vi "TSP-Link Reset.vi"(8 "error in (no error)":errorcluster, 11 "VISA resource name":refnum<visa-resource-name>) -> (0 "error out":errorcluster, 3 "VISA resource name out":refnum<visa-resource-name>, 4 "Command String":string)   [LabVIEW 2012, in "Keithley 2600 Series.lvlib"]
doc: "Initializes (resets) all nodes (instruments) in the TSP-Link system.\n\nThis VI will erase all knowledge of other nodes connected on the TSP-Link and will regenerate the system configuration. This VI must be called at least once before any remote nodes can be accessed. If the node number for any instrument is changed, the TSP-Link must again be initialized.\n\n<b>Functions and Attributes Used</b>\ntsplink.reset()\n\nNote:\nTSP-Link feature is not supported with Keithley 2604B, 2614B, 2634B."
uses:
  Keithley 2600 Series.lvlib
  Private/GlobalVariables.vi
panel:
  # "(c) 2008 Keithley Instruments, Inc.  ALL RIGHTS RESERVED."
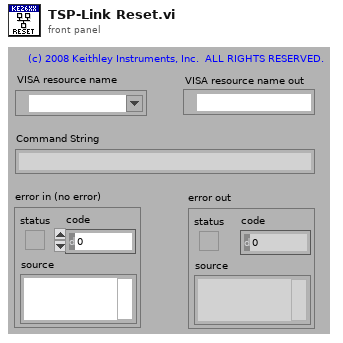
[diagram p1: front panel]
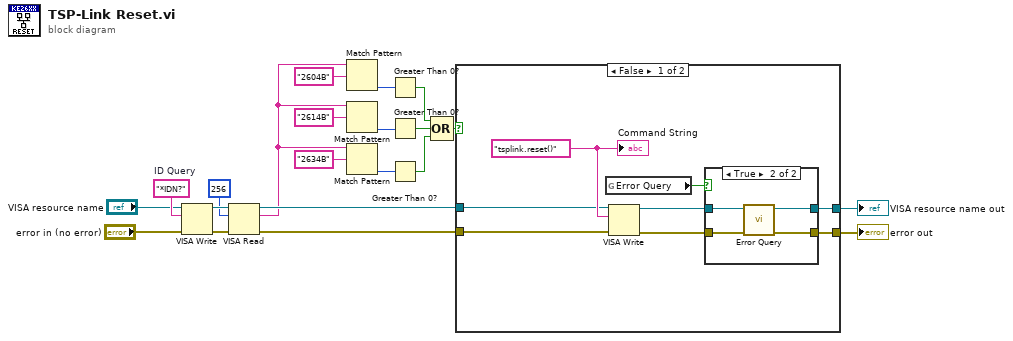
[diagram p0: block diagram]
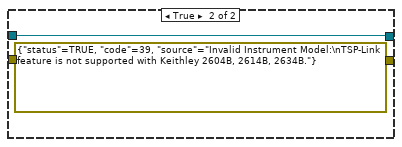
[diagram p3: hidden frame]
diagram:
  w16 = "*IDN?"  # ID Query
  n1 = VISA Write(VISA resource name="VISA resource name", write buffer=w16, error in (no error)="error in (no error)") -> (VISA resource name out=w19:refnum<visa-resource-name>, error out=w18:errorcluster)  [unwired: 1 out]
  n2 = VISA Read(VISA resource name=w19, byte count=u32 256, error in (no error)=w18) -> (VISA resource name out=w13:refnum<visa-resource-name>, read buffer=w2:string, error out=w12:errorcluster)  [unwired: 1 out]
  n3 = Match Pattern(string=w2, regular expression="2604B" ("y")) -> (offset past match=w8:i32)  [unwired: 1 in, 3 out]
  n4 = Match Pattern(string=w2, regular expression="2614B" ("y")) -> (offset past match=w7:i32)  [unwired: 1 in, 3 out]
  n5 = Match Pattern(string=w2, regular expression="2634B" ("y")) -> (offset past match=w6:i32)  [unwired: 1 in, 3 out]
  n6 = Greater Than 0?(x=w8) -> (x > 0?=w5:bool)
  n7 = Greater Than 0?(x=w7) -> (x > 0?=w4:bool)
  n8 = Greater Than 0?(x=w6) -> (x > 0?=w3:bool)
  n9 = Compound Arithmetic op=OR(w5, w4, w3) -> (w1:bool)
  n10 = case shown="False" w1 {
    tunnel: [w25 w37] -> w21
    tunnel: [w24 errorcluster {"status"=TRUE, "code"=39, "source"="Invalid Instrument Model:\nTSP-Link feature is not supported with Keithley 2604B, 2614B, 2634B."} ("error out")] -> w20
    tunnel: w13 -> [w23 w37]
    tunnel: w12 -> [w22 _]
    frame False {
      w29 = "tsplink.reset()" ("command")
      n11 = global read "GlobalVariables.vi" "Error Query"() -> (w28:bool)
      n12 = VISA Write(VISA resource name=w23, write buffer=w29, error in (no error)=w22) -> (VISA resource name out=w27:refnum<visa-resource-name>, error out=w26:errorcluster)  [unwired: 1 out]
      n13 = case shown="True" w28 {
        tunnel: w27 -> [w31 w35]
        tunnel: w26 -> [w30 w34]
        tunnel: [w31 w33] -> w25
        tunnel: [w30 w32] -> w24
        frame False {
        }
        frame True {
          n14 = call "Error Query.vi"("error in (no error)"=w34, "VISA resource name"=w35) -> ("error out"=w32:errorcluster, "VISA resource name out"=w33:refnum<visa-resource-name>)  [unwired: 8 out]
        }
      }
      "Command String" <- w29
    }
    frame True {
    }
  }
  "VISA resource name out" <- w21
  "error out" <- w20
